vi "model.vi"() -> ()   [LabVIEW 2017]
panel:
  out "Waveform Chart":dbl(graph)
  in  "steps":i32
  in  "SNRs":dbl[](array[numeric])
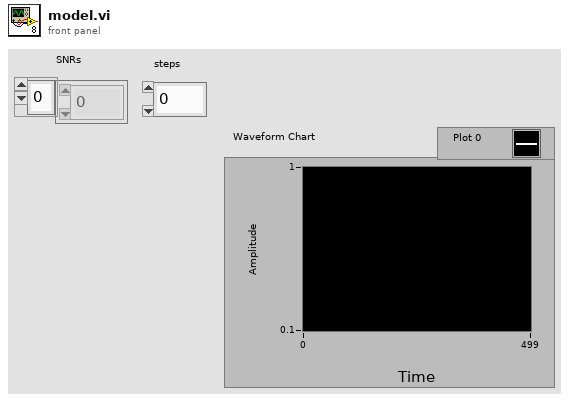
[diagram p1: front panel]
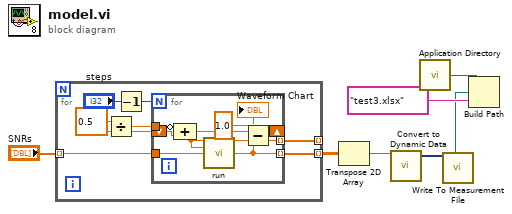
[diagram p0: block diagram]
diagram:
  n1 = for {
    tunnel: "SNRs" -> [w12] mode=indexing
    tunnel: [w9] -> w1 mode=indexing
    tunnel: [w8] -> _ mode=indexing
    w13 = 0.5
    n2 = Divide(x=w13, y="steps") -> (x/y=w14:dbl)
    n3 = Decrement(x="steps") -> (x-1=w10:i32)
    n4 = for {
      N: w10 -> [_]
      tunnel: w14 -> [w22]
      shift-right: [w20] -> _
      shift-left: w13 -> [w21]
      tunnel: w12 -> [w19]
      tunnel: [w15] -> w9 mode=indexing
      tunnel: [w16] -> w8 mode=indexing
      n5 = Compound Arithmetic op=ADD(invert w22, w21) -> (w20:dbl)
      n6 = call "run.vi"("p12"=w20, "p21"=w20, "SNR"=w19) -> ("p12"=w18:dbl, "p"=w15:dbl)  [unwired: 11 in]
      "Waveform Chart" <- w15
      n7 = Subtract(x=1.0, y=w18) -> (x-y=w16:dbl)
    }
  }
  n8 = Transpose 2D Array(2D array=w1) -> (transposed array=w6:dbl[][])
  n9 = call "Convert to Dynamic Data"("2D Array"=w6) -> ("Dynamic Data Type"=w5:dynamicdata)  [unwired: 3 in]
  n10 = call <vilib>:"Application Directory.vi"() -> ("Application Directory"=w2:path)
  n11 = Build Path(base path=w2, name or relative path="test3.xlsx") -> (appended path=w3:path)
  n12 = call "Write To Measurement File"("Signals"=w5, "Filename"=w3) -> ()  [unwired: 15 in, 3 out]
